vi "Parse DIO64.vi"(7 "error in":errorcluster, 8 "recusion depth":i32=100, 9 "DIO64":T2(array[cluster]) {"end time" format="%#_8g"; "begin time" format="%#_8g"}) -> (0 "error out":errorcluster, 2 "times":T1(array[cluster]) {"end time" format="%#_8g"; "begin time" format="%#_8g"})   [LabVIEW 2012]
uses:
  <vilib>/Utility/error.llb/DialogType.ctl
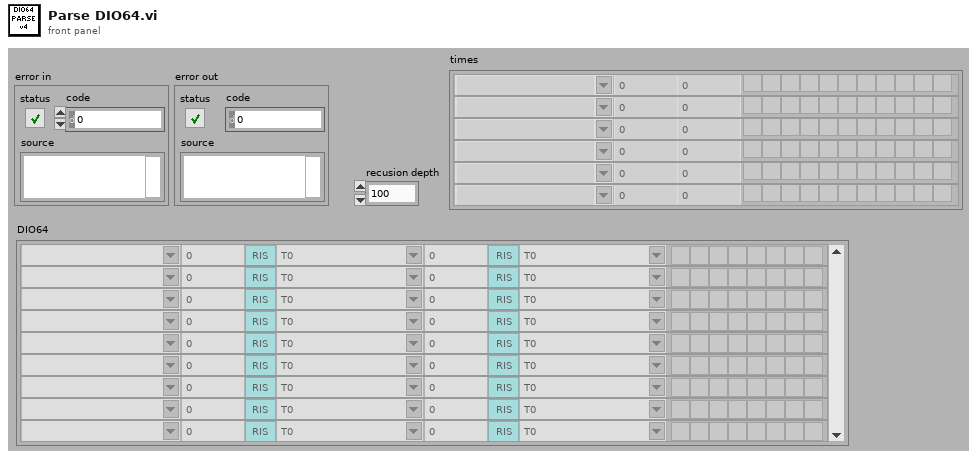
[diagram p1: front panel]
types:
  T1 = cluster{"Task":string, "begin time":dbl, "end time":dbl, "Chops":bool[]}[]
  T2 = cluster{"Task":string, "begin time":dbl, "begin edge":bool, "begin reference":string, "end time":dbl, "end edge":bool, "end reference":string, "Chops":bool[]}[]
  T3 = cluster{"Task":string, "begin time":dbl, "end time":dbl, "chops":bool[]}
  T4 = cluster{"Task":string, "begin time":dbl, "begin edge":bool, "begin reference":string, "end time":dbl, "end edge":bool, "end reference":string, "Chops":bool[]}
  T5 = cluster{"Task":string, "begin time":dbl, "end time":dbl, "chops":bool[]}[]
  T6 = typedef "DialogType.ctl" = u16
  T7 = cluster{"begin time":dbl, "Task":string, "end time":dbl, "chops":bool[]}
  T8 = cluster{"begin time":dbl, "Task":string, "end time":dbl, "chops":bool[]}[]
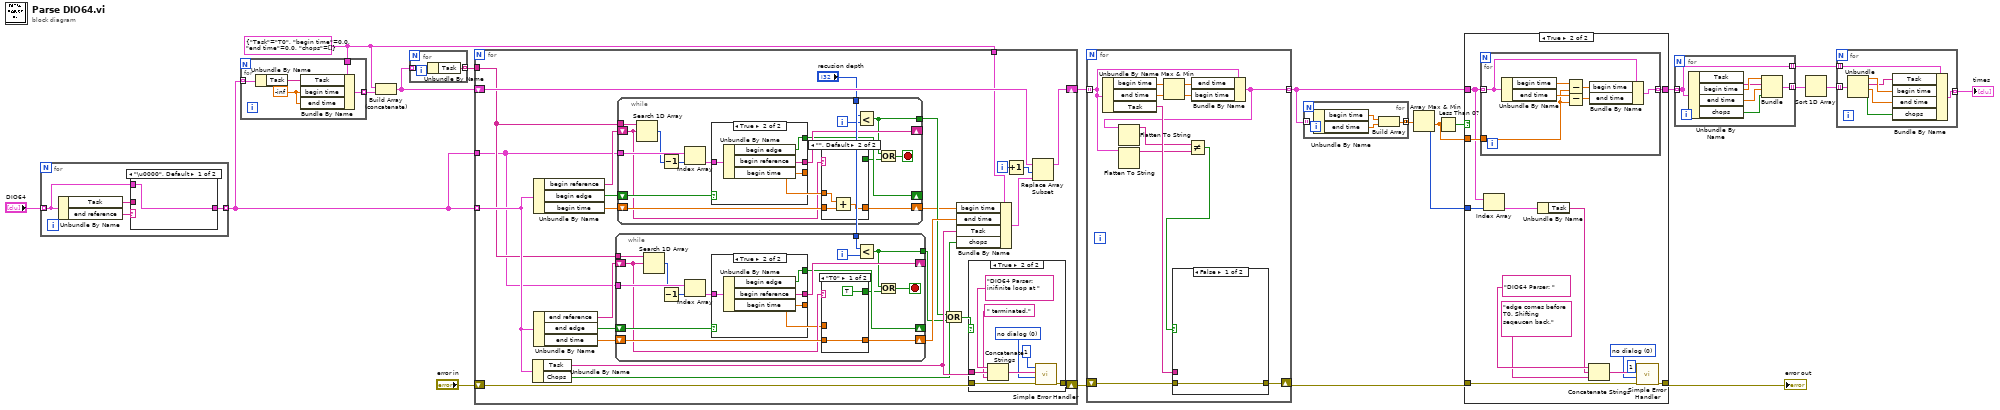
[diagram p0: block diagram]
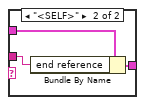
[diagram p2: hidden frame]
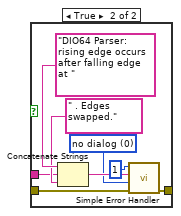
[diagram p4: hidden frame]
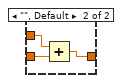
[diagram p6: hidden frame]
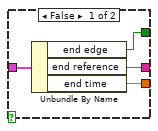
[diagram p7: hidden frame]
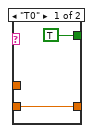
[diagram p8: hidden frame]
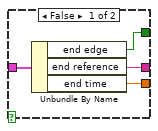
[diagram p9: hidden frame]
diagram:
  w3 = T3 {"Task"="T0", "begin time"=0.0, "end time"=0.0, "chops"=[]} ("Task")
  n1 = for {
    tunnel: "DIO64" -> [w24] mode=indexing
    tunnel: [w22] -> w1 mode=indexing
    n2 = Unbundle By Name(w24) -> ("Task"=w23:string, "end reference"=w25:string)
    n3 = case shown="\"\", Default" w25 {
      tunnel: w24 -> [w26 w29]
      tunnel: w23 -> [_ w28]
      tunnel: [w26 w27] -> w22
      frame "\u0000", Default {
      }
      frame "<SELF>" {
        n4 = Bundle By Name(cluster=w29, "end reference"=w28) -> (w27:T4)
      }
    }
  }
  n5 = for {
    tunnel: w1 -> [w34] mode=indexing
    tunnel: w3 -> [w33]
    tunnel: [w31] -> w21 mode=indexing
    w30 = -inf
    n6 = Unbundle By Name(w34) -> ("Task"=w32:string)
    n7 = Bundle By Name(cluster=w33, "Task"=w32, "begin time"=w30, "end time"=w30) -> (w31:T3)
  }
  n8 = Build Array (concatenate)(w3, w21) -> (w20:T5)
  n9 = for {
    tunnel: w20 -> [w36] mode=indexing
    tunnel: [w35] -> w19 mode=indexing
    n10 = Unbundle By Name(w36) -> ("Task"=w35:string)
  }
  n11 = for {
    shift-right: [w57] -> w5
    shift-left: w20 -> [w54]
    tunnel: w1 -> [w50] mode=indexing
    tunnel: w19 -> [w49]
    tunnel: w1 -> [w48]
    shift-right: [w45] -> w18
    shift-left: "error in" -> [w44]
    tunnel: w3 -> [w38]
    i -> [w56]
    n12 = Unbundle By Name(w50) -> ("Task"=w43:string, "Chops"=w39:bool[])
    n13 = Unbundle By Name(w50) -> ("begin reference"=w61:string, "begin edge"=w60:bool, "begin time"=w59:dbl)
    n14 = Unbundle By Name(w50) -> ("end reference"=w51:string, "end edge"=w52:bool, "end time"=w53:dbl)
    n15 = while {
      tunnel: w49 -> [w87]
      shift-right: [w82] -> _
      shift-left: w51 -> [w76]
      shift-right: [w84] -> w47
      shift-left: w53 -> [w85]
      tunnel: w48 -> [w83]
      shift-right: [w81] -> _
      shift-left: w52 -> [w86]
      tunnel: "recusion depth" -> [w78]
      tunnel: [w77] -> w40
      i -> [w79]
      stop <- w80 stop-if-true
      n16 = Search 1D Array(1D array=w87, element=w76) -> (index of element=w72:i32)  [unwired: 1 in]
      n17 = Decrement(x=w72) -> (x-1=w73:i32)
      n18 = Index Array(array=w83, index=w73) -> (element=w75:T4)
      n19 = case shown="True" w86 {
        tunnel: w75 -> [w96 w100]
        tunnel: [w95 w99] -> w74
        tunnel: [w94 w98] -> w82
        tunnel: [w93 w97] -> w81
        frame False {
          n20 = Unbundle By Name(w96) -> ("end edge"=w93:bool, "end reference"=w94:string, "end time"=w95:dbl)
        }
        frame True {
          n21 = Unbundle By Name(w100) -> ("begin edge"=w97:bool, "begin reference"=w98:string, "begin time"=w99:dbl)
        }
      }
      n22 = case shown="\"T0\"" w76 {
        tunnel: w85 -> [w89 w91]
        tunnel: [w89 w92] -> w84
        tunnel: w74 -> [_ w90]
        tunnel: [TRUE _] -> w71
        frame "T0" {
        }
        frame "", Default {
          n23 = Add(x=w90, y=w91) -> (x+y=w92:dbl)
        }
      }
      n24 = Less?(x=w78, y=w79) -> (x < y?=w77:bool)
      n25 = Or(x=w77, y=w71) -> (x .or. y?=w80:bool)
    }
    n26 = while {
      tunnel: w49 -> [w117]
      shift-right: [w108] -> _
      shift-left: w61 -> [w105]
      shift-right: [w114] -> w37
      shift-left: w59 -> [w115]
      tunnel: w48 -> [w113]
      shift-right: [w107] -> _
      shift-left: w60 -> [w116]
      tunnel: "recusion depth" -> [w102]
      tunnel: [w101] -> w41
      i -> [w103]
      stop <- w106 stop-if-true
      n27 = Search 1D Array(1D array=w117, element=w105) -> (index of element=w109:i32)  [unwired: 1 in]
      n28 = Decrement(x=w109) -> (x-1=w110:i32)
      n29 = Index Array(array=w113, index=w110) -> (element=w112:T4)
      n30 = case shown="True" w116 {
        tunnel: w112 -> [w126 w130]
        tunnel: [w125 w129] -> w111
        tunnel: [w124 w128] -> w108
        tunnel: [w123 w127] -> w107
        frame False {
          n31 = Unbundle By Name(w126) -> ("end edge"=w123:bool, "end reference"=w124:string, "end time"=w125:dbl)
        }
        frame True {
          n32 = Unbundle By Name(w130) -> ("begin edge"=w127:bool, "begin reference"=w128:string, "begin time"=w129:dbl)
        }
      }
      n33 = case shown="\"\", Default" w105 {
        tunnel: w115 -> [w119 w121]
        tunnel: [w119 w122] -> w114
        tunnel: w111 -> [_ w120]
        tunnel: [TRUE _] -> w104
        frame "T0" {
        }
        frame "", Default {
          n34 = Add(x=w120, y=w121) -> (x+y=w122:dbl)
        }
      }
      n35 = Less?(x=w102, y=w103) -> (x < y?=w101:bool)
      n36 = Or(x=w101, y=w104) -> (x .or. y?=w106:bool)
    }
    n37 = Or(x=w41, y=w40) -> (x .or. y?=w42:bool)
    n38 = Bundle By Name(cluster=w38, "begin time"=w37, "end time"=w47, "Task"=w43, "chops"=w39) -> (w58:T3)
    n39 = case shown="True" w42 {
      tunnel: [w62 w70] -> w45
      tunnel: w44 -> [w62 w69]
      tunnel: w43 -> [_ w67]
      frame False {
      }
      frame True {
        w63 = T6 0 items=["no dialog", "OK message", "continue or stop message", "OK message + warnings", "continue/stop + warnings"] ("type of dialog (OK msg:1)")
        n40 = Concatenate Strings("DIO64 Parser: inifinite loop at " ("string"), w67, " terminated." ("string")) -> (w68:string)
        n41 = call <vilib>:"Simple Error Handler.vi"("error code (no error:0)"=1, "error source (\" \")"=w68, "type of dialog (OK msg:1)"=w63, "error in (no error)"=w69) -> ("error out"=w70:errorcluster)  [unwired: 1 in, 4 out]
      }
    }
    n42 = Increment(x=w56) -> (x+1=w55:i32)
    n43 = Replace Array Subset(array=w54, new element=w58, index=w55) -> (w57:T5)
  }
  n44 = for {
    tunnel: w5 -> [w134] mode=indexing
    tunnel: [w135] -> w4 mode=indexing
    shift-right: [w136] -> w14
    shift-left: w18 -> [w137]
    n45 = Unbundle By Name(w134) -> ("begin time"=w141:dbl, "end time"=w142:dbl, "Task"=w138:string)
    n46 = Flatten To String(anything=w134) -> (data string=w132:string)  [unwired: 3 in, 2 out]
    n47 = Max & Min(x=w141, y=w142) -> (max(x,y)=w140:dbl, min(x,y)=w139:dbl)
    n48 = Bundle By Name(cluster=w134, "end time"=w140, "begin time"=w139) -> (w135:T3)
    n49 = Flatten To String(anything=w135) -> (data string=w133:string)  [unwired: 3 in, 2 out]
    n50 = Not Equal?(x=w133, y=w132) -> (x != y?=w131:bool)
    n51 = case shown="False" w131 {
      tunnel: [w143 w151] -> w136
      tunnel: w138 -> [_ w145]
      tunnel: w137 -> [w143 w144]
      frame False {
      }
      frame True {
        w146 = T6 0 items=["no dialog", "OK message", "continue or stop message", "OK message + warnings", "continue/stop + warnings"] ("type of dialog (OK msg:1)")
        n52 = Concatenate Strings("DIO64 Parser: rising edge occurs after falling edge at " ("string"), w145, " . Edges swapped." ("string")) -> (w150:string)
        n53 = call <vilib>:"Simple Error Handler.vi"("error code (no error:0)"=1, "error source (\" \")"=w150, "type of dialog (OK msg:1)"=w146, "error in (no error)"=w144) -> ("error out"=w151:errorcluster)  [unwired: 1 in, 4 out]
      }
    }
  }
  n54 = for {
    tunnel: w4 -> [w155] mode=indexing
    tunnel: [w152] -> w17 mode=concatenating
    n55 = Unbundle By Name(w155) -> ("begin time"=w154:dbl, "end time"=w153:dbl)
    n56 = Build Array(w154, w153) -> (w152:dbl[])
  }
  n57 = Array Max & Min(array=w17) -> (min value=w15:dbl, min index (indices)=w12:i32)  [unwired: 2 out]
  n58 = Less Than 0?(x=w15) -> (x < 0?=w16:bool)
  n59 = case shown="True" w16 {
    tunnel: w15 -> [_ w170]
    tunnel: w4 -> [w157 w160]
    tunnel: [w157 w169] -> w11
    tunnel: w14 -> [w156 w163]
    tunnel: [w156 w162] -> w13
    tunnel: w12 -> [_ w161]
    frame False {
    }
    frame True {
      w164 = T6 0 items=["no dialog", "OK message", "continue or stop message", "OK message + warnings", "continue/stop + warnings"] ("type of dialog (OK msg:1)")
      n60 = for {
        tunnel: w160 -> [w177] mode=indexing
        tunnel: w170 -> [w174]
        tunnel: [w171] -> w169 mode=indexing
        n61 = Unbundle By Name(w177) -> ("begin time"=w176:dbl, "end time"=w175:dbl)
        n62 = Subtract(x=w176, y=w174) -> (x-y=w173:dbl)
        n63 = Subtract(x=w175, y=w174) -> (x-y=w172:dbl)
        n64 = Bundle By Name(cluster=w177, "begin time"=w173, "end time"=w172) -> (w171:T3)
      }
      n65 = Index Array(array=w160, index=w161) -> (element=w159:T3)
      n66 = Unbundle By Name(w159) -> ("Task"=w158:string)
      n67 = Concatenate Strings("DIO64 Parser: " ("string"), w158, "edge comes before T0. Shifting seqeucen back." ("string")) -> (w168:string)
      n68 = call <vilib>:"Simple Error Handler.vi"("error code (no error:0)"=1, "error source (\" \")"=w168, "type of dialog (OK msg:1)"=w164, "error in (no error)"=w163) -> ("error out"=w162:errorcluster)  [unwired: 1 in, 4 out]
    }
  }
  "error out" <- w13
  n69 = for {
    tunnel: w11 -> [w179] mode=indexing
    tunnel: [w180] -> w10 mode=indexing
    tunnel: [w179] -> w8 mode=indexing
    n70 = Unbundle By Name(w179) -> ("Task"=w182:string, "begin time"=w183:dbl, "end time"=w181:dbl, "chops"=w178:bool[])
    n71 = Bundle("begin time"=w183, "Task"=w182, "end time"=w181, "chops"=w178) -> (w180:T7)  [unwired: 1 in]
  }
  n72 = Sort 1D Array(array=w10) -> (sorted array=w9:T8)
  n73 = for {
    tunnel: w9 -> [w190] mode=indexing
    tunnel: w8 -> [w189] mode=indexing
    tunnel: [w185] -> w7 mode=indexing
    n74 = Unbundle(w190) -> ("begin time"=w188:dbl, "Task"=w187:string, "end time"=w186:dbl, "chops"=w184:bool[])
    n75 = Bundle By Name(cluster=w189, "Task"=w187, "begin time"=w188, "end time"=w186, "chops"=w184) -> (w185:T3)
  }
  "times" <- w7
